vi "GE hWnd Handler.vi"(7 "This VI":refnum<vi>, 8 "error in":errorcluster, 11 "Refnum In":refnum<k7>) -> (0 "error out":errorcluster, 3 "Refnum Out":refnum<k7>)   [LabVIEW 8.6]
uses:
  user32.dll
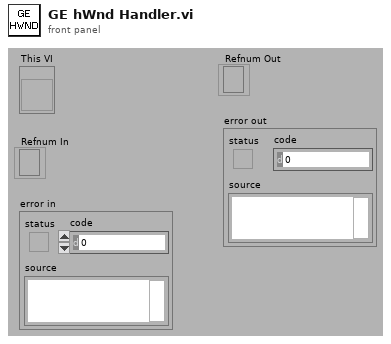
[diagram p1: front panel]
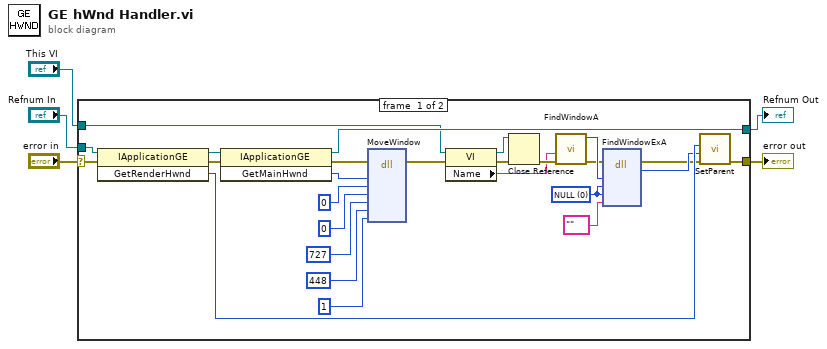
[diagram p0: block diagram]
diagram:
  n1 = case shown="No Error" "error in" {
    selector: "error in" -> [w6 w33]
    tunnel: "Refnum In" -> [w29 w32]
    tunnel: [w28 w32] -> w4
    tunnel: "This VI" -> [w18 _]
    tunnel: [w16 w33] -> w2
    frame #0 {
      w17 = 0 items=["NULL"]
      n2 = invoke class="IApplicationGE" method="GetRenderHwnd"(reference=w29, error in=w6) -> (reference out=w27:refnum<k7>, error out=w26:errorcluster, "GetRenderHwnd"=w31:i32)  [unwired: 1 in]
      n3 = invoke class="IApplicationGE" method="GetMainHwnd"(reference=w27, error in=w26) -> (reference out=w28:refnum<k7>, error out=w25:errorcluster, "GetMainHwnd"=w24:i32)  [unwired: 1 in]
      n4 = dll-call lib="user32.dll" fn="MoveWindow"(error in=w25, "hWnd"=w24, "X"=u32 0, "Y"=0, "nWidth"=u32 727, "nHeight"=u32 448, "bRepaint"=u8 1) -> (error out=w30:errorcluster)  [unwired: 5 in, 5 out]
      n5 = property class="VI"(reference=w18, error in=w30) -> (reference out=w15:refnum<vi>, error out=w14:errorcluster, "Name"=w9:string)
      n6 = Close Reference(reference=w15, error in (no error)=w14) -> (error out=w10:errorcluster)
      n7 = call "FindWindowA.vi"("error in"=w10, "lpszWindowName"=w9) -> ("error out"=w7:errorcluster, "hWnd"=w8:u32)  [unwired: 6 in, 2 out]
      n8 = dll-call lib="user32.dll" fn="FindWindowExA"(error in=w7, "Parent HWND"=w8, "Child_After HWND"=w17, "lpszClassName"=w17, "lpszWindowName"="") -> (error out=w12:errorcluster, "hWnd"=w13:u32)  [unwired: 5 in, 2 out]
      n9 = call "SetParent.vi"("error in"=w12, "hWndNewParent"=w13, "hWndChild"=w31) -> ("error out"=w16:errorcluster)  [unwired: 5 in, 3 out]
    }
    frame #1 {
    }
  }
  "Refnum Out" <- w4
  "error out" <- w2
